vi "SetValue.vi"(10 "cluster":T1, 11 "TaskConfig":T2={"Drive"=enum."NI_DAQmx", "TaskType"=enum."AI", "PhysicalChannels"="/Dev1/ai0:3", "SampleRateConfiguration"={"SampleRate"=1000.0, "SamplesPerChannel"=1000, "SamplesPerRead"=200, "SampleMode"=10123, "Clock Source"="OnboardClock"}, "ChannelConfig"={}, "Enable"=FALSE, "ShowPanel"=FALSE} {"SampleRateConfiguration"."SampleMode" items=["Finite Samples"=10178, "Continuous Samples"=10123, "Hardware Timed Single Point"=12522]}) -> ()   [LabVIEW 2025, in "DAQ_Module.lvlib" / "DAQ_Module.lvclass"]
uses:
  DAQ_Module.lvclass
  DAQ_Task_Config.ctl
  DAQ_HW_Type.ctl
  DAQ_Task_Type.ctl
  DAQ_SampleRateConfig.ctl
  DAQ_Task_UIobject.ctl
  DAQ_Module.lvclass/DAQ_Module.ctl
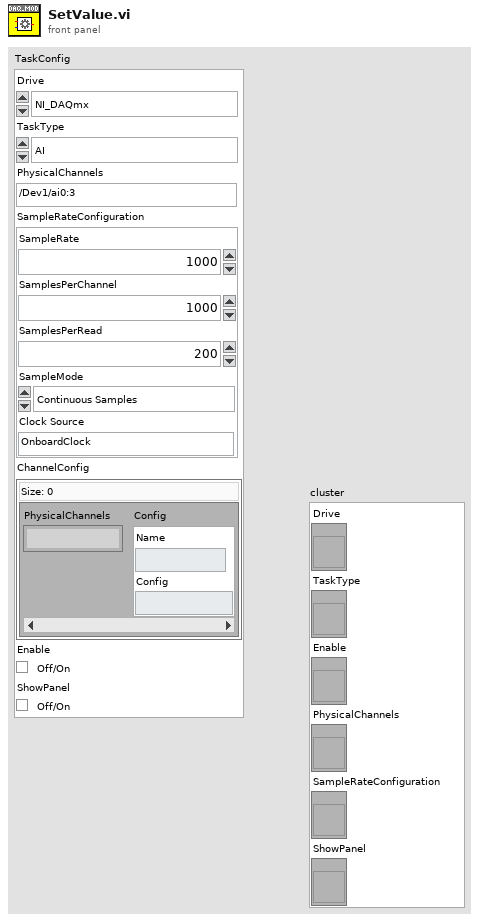
[diagram p1: front panel]
types:
  T1 = typedef "DAQ_Module.lvlib/DAQ_Module.lvclass/DAQ_Task_UIobject.ctl" = cluster{"Drive":refnum<vi>, "TaskType":refnum<vi>, "Enable":refnum<vi>, "PhysicalChannels":refnum<vi>, "SampleRateConfiguration":refnum<vi>, "ShowPanel":refnum<vi>}
  T2 = typedef "DAQ_Module.lvlib/DAQ_Module.lvclass/DAQ_Task_Config.ctl" = cluster{"Drive":T3, "TaskType":T4, "PhysicalChannels":string, "SampleRateConfiguration":T5, "ChannelConfig":map{string, cluster{"Name":string, "Config":string}}, "Enable":bool, "ShowPanel":bool}
  T3 = typedef "DAQ_Module.lvlib/DAQ_Module.lvclass/DAQ_HW_Type.ctl" = enum16{"NI_DAQmx", "Simulated_DAQ"}
  T4 = typedef "DAQ_Module.lvlib/DAQ_Module.lvclass/DAQ_Task_Type.ctl" = enum16{"AI", "Linear", "Angular", "AO"}
  T5 = typedef "DAQ_Module.lvlib/DAQ_Module.lvclass/DAQ_SampleRateConfig.ctl" = cluster{"SampleRate":dbl, "SamplesPerChannel":u32, "SamplesPerRead":i32, "SampleMode":i32, "Clock Source":string}
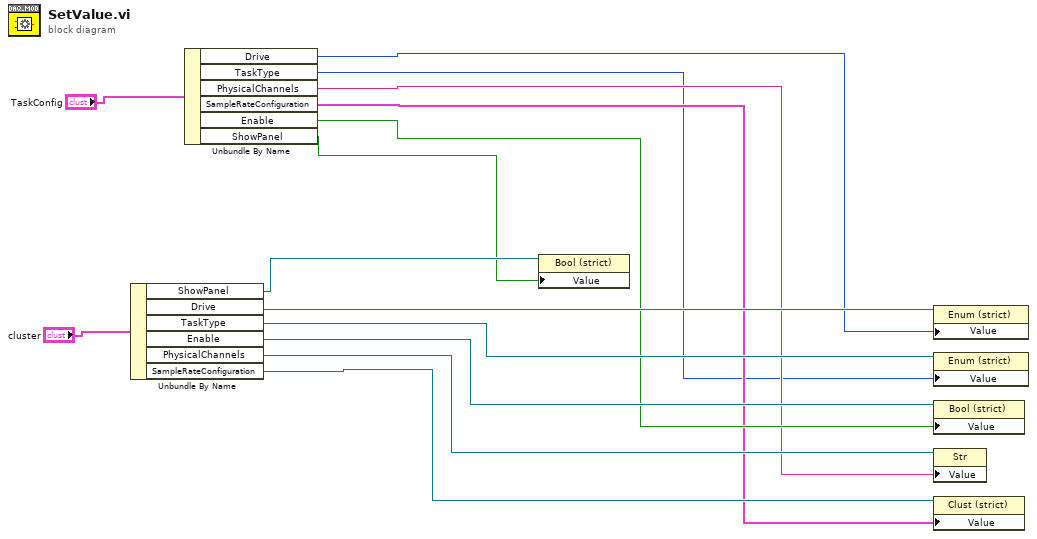
[diagram p0: block diagram]
diagram:
  n1 = Unbundle By Name("cluster") -> ("ShowPanel"=w2:refnum<vi>, "Drive"=w14:refnum<vi>, "TaskType"=w13:refnum<vi>, "Enable"=w12:refnum<vi>, "PhysicalChannels"=w11:refnum<vi>, "SampleRateConfiguration"=w10:refnum<vi>)
  n2 = Unbundle By Name("TaskConfig") -> ("Drive"=w7:T3, "TaskType"=w3:T4, "PhysicalChannels"=w5:string, "SampleRateConfiguration"=w4:T5, "Enable"=w6:bool, "ShowPanel"=w1:bool)
  n3 = property class="Bool (strict)"(reference=w2, "Value"=w1) -> ()  [unwired: 1 in, 2 out]
  n4 = property class="Enum (strict)"(reference=w14, "Value"=w7) -> ()  [unwired: 1 in, 2 out]
  n5 = property class="Enum (strict)"(reference=w13, "Value"=w3) -> ()  [unwired: 1 in, 2 out]
  n6 = property class="Bool (strict)"(reference=w12, "Value"=w6) -> ()  [unwired: 1 in, 2 out]
  n7 = property class="Str"(reference=w11, "Value"=w5) -> ()  [unwired: 1 in, 2 out]
  n8 = property class="Clust (strict)"(reference=w10, "Value"=w4) -> ()  [unwired: 1 in, 2 out]
